vi "Image_RAW_Get_Frame.vi"(8 "error in (no error)":errorcluster, 9 "Bytes per Frame":u32, 11 "RAW refnum In":refnum<file>) -> (0 "error out":errorcluster, 2 "Frame (U8)":u8[](array[numeric]), 3 "RAW refnum Out":refnum<file>)   [LabVIEW 2020]
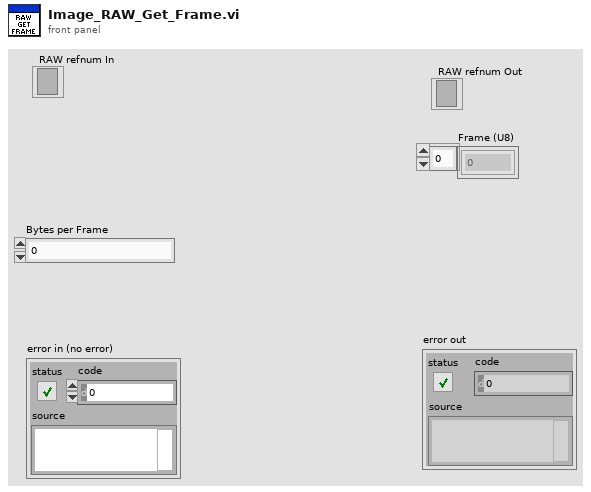
[diagram p1: front panel]
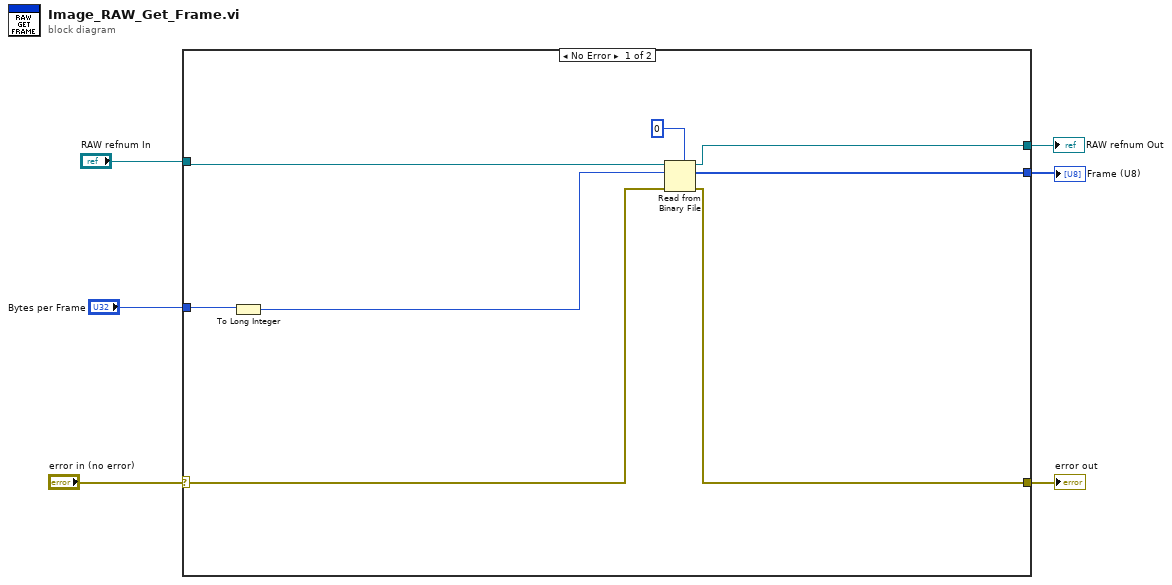
[diagram p0: block diagram]
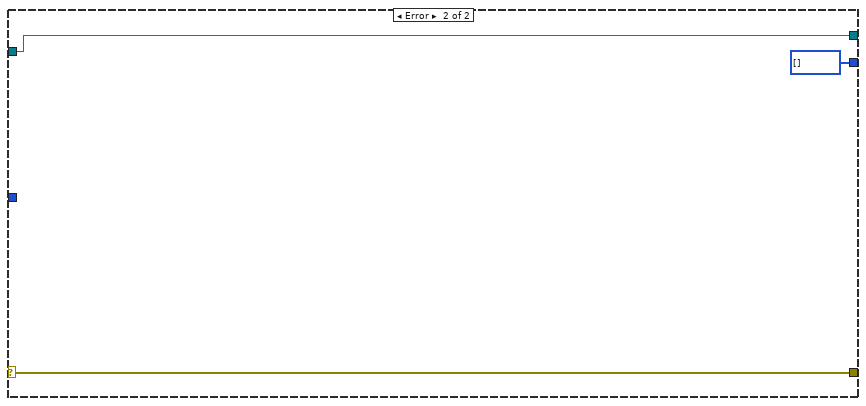
[diagram p2: hidden frame]
diagram:
  n1 = case shown="No Error" "error in (no error)" {
    selector: "error in (no error)" -> [w7 w16]
    tunnel: "RAW refnum In" -> [w10 w17]
    tunnel: "Bytes per Frame" -> [w9 _]
    tunnel: [w13 w17] -> w3
    tunnel: [w12 w16] -> w2
    tunnel: [w11 u8[] []] -> w1
    frame No Error {
      n2 = To Long Integer(number=w9) -> (32bit integer=w8:i32)
      n3 = Read from Binary File(5:u8 0, 8:w7, 10:w8, 11:w10) -> (0:w12:errorcluster, 2:w11:u8[], 3:w13:refnum<file>)  [unwired: 2 in, 1 out]
    }
    frame Error {
    }
  }
  "error out" <- w2
  "RAW refnum Out" <- w3
  "Frame (U8)" <- w1
